vi "test_DAC_IO.vi"() -> ()   [LabVIEW 2019]
uses:
  <vilib>/DAQmx/write.llb/DAQmx Write (Analog Wfm 1Chan NSamp).vi
  <vilib>/DAQmx/read.llb/DAQmx Read (Analog DBL 1Chan 1Samp).vi
  <vilib>/DAQmx/create/channels.llb/DAQmx Create Channel (AO-Voltage-Basic).vi
  <vilib>/DAQmx/configure/timing.llb/DAQmx Timing (Use Waveform).vi
  <vilib>/DAQmx/miscellaneous.llb/DAQmx Fill In Error Info.vi
  <vilib>/DAQmx/create/channels.llb/DAQmx Create Channel (AI-Voltage-Basic).vi
  <vilib>/DAQmx/configure/timing.llb/DAQmx Timing (Sample Clock).vi
panel:
  in  "auto_stop":bool
  in  "stop":bool
  out "wf_chart_in":dbl(graph)
  in  "rate_in":dbl=1000.0 format="%0.2f"
  in  "chan_in":tag
  out "message":string
  out "wf_graph_out":waveform(dbl)(graph)
  in  "waveform":T1(ring)
  in  "N_steps":i32=100
  in  "T_sweep":dbl=1.0
  in  "N_sweeps":i32=2
  in  "chan_out":tag="Dev1/ao0"
  # "s"
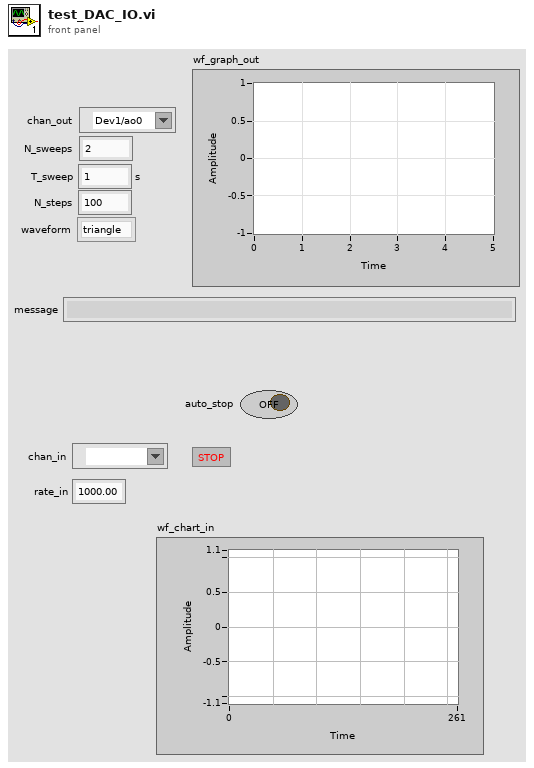
[diagram p1: front panel]
types:
  T1 = enum16{"triangle", "saw_direct", "saw_invert", "sine"}
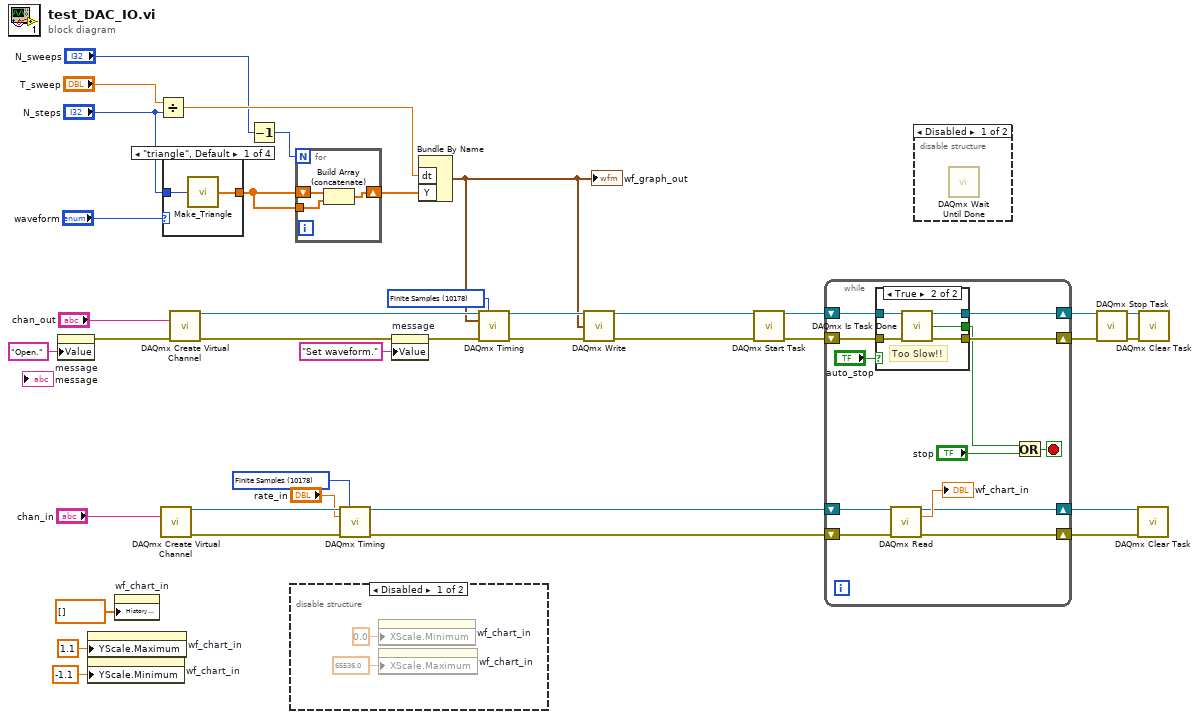
[diagram p0: block diagram]
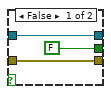
[diagram p4: hidden frame]
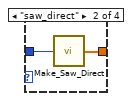
[diagram p5: hidden frame]
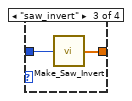
[diagram p6: hidden frame]
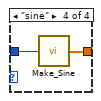
[diagram p7: hidden frame]
diagram:
  w11 = 10178 items=["Finite Samples"=10178, "Continuous Samples"=10123, "Hardware Timed Single Point"=12522] ("sample mode")
  w38 = 10178 items=["Finite Samples"=10178, "Continuous Samples"=10123, "Hardware Timed Single Point"=12522] ("sample mode")
  n1 = property on="message" class="Str"("Value"="Open." ("message")) -> (error out=w22:errorcluster)  [unwired: 2 in, 1 out]
  n2 = property on="wf_chart_in" class="WFChart (strict)"("YScale.Maximum"=1.1 ("Y Scale.Range:Maximum")) -> ()  [unwired: 2 in, 2 out]
  n3 = property on="wf_chart_in" class="WFChart (strict)"("YScale.Minimum"=-1.1 ("Y Scale.Range:Minimum")) -> ()  [unwired: 2 in, 2 out]
  n4 = property on="wf_chart_in" class="WFChart (strict)"("History Data"=dbl[] []) -> ()  [unwired: 2 in, 2 out]
  n5 = Divide(x="T_sweep", y="N_steps") -> (x/y=w29:dbl)
  n6 = call-poly <vilib>:"DAQmx Create Virtual Channel.vi"("physical channels"="chan_in") -> ("task out"=w15:refnum<k21>, "error out"=w13:errorcluster)  [unwired: 13 in]
  n7 = case shown="\"triangle\", Default" "waveform" {
    tunnel: "N_steps" -> [w41 w43 w45 w47]
    tunnel: [w40 w42 w44 w46] -> w30
    frame "triangle", Default {
      n8 = call "Make_Triangle.vi"("N_steps_1"=w41) -> ("TriangleWaveform"=w40:dbl[])
    }
    frame "saw_direct" {
      n9 = call "Make_Saw_Direct.vi"("N_steps_1"=w43) -> ("SawDirectWaveform"=w42:dbl[])
    }
    frame "saw_invert" {
      n10 = call "Make_Saw_Invert.vi"("N_steps_1"=w45) -> ("SawInvertWaveform"=w44:dbl[])
    }
    frame "sine" {
      n11 = call "Make_Sine.vi"("N_steps_1"=w47) -> ("SineWaveform"=w46:dbl[])
    }
  }
  n12 = call-poly <vilib>:"DAQmx Create Virtual Channel.vi"("physical channels"="chan_out", "error in"=w22) -> ("task out"=w32:refnum<k21>, "error out"=w20:errorcluster)  [unwired: 12 in]
  n13 = Decrement(x="N_sweeps") -> (x-1=w28:i32)
  n14 = disable-structure shown="Disabled" {
    frame Disabled {
      n15 = property on="wf_chart_in" class="WFChart (strict)"("XScale.Minimum"=0.0 ("X Scale.Range:Minimum")) -> ()  [unwired: 2 in, 2 out]
      n16 = property on="wf_chart_in" class="WFChart (strict)"("XScale.Maximum"=65536.0 ("X Scale.Range:Maximum")) -> ()  [unwired: 2 in, 2 out]
    }
    frame Enabled {
    }
  }
  n17 = for {
    N: w28 -> [_]
    shift-right: [w50] -> w31
    shift-left: w30 -> [w52]
    tunnel: w30 -> [w51]
    n18 = Build Array (concatenate)(w52, w51) -> (w50:dbl[])
  }
  n19 = call-poly <vilib>:"DAQmx Timing.vi"("task/channels in"=w15, "sample mode"=w11, "rate"="rate_in", "error in"=w13) -> ("task out"=w14:refnum<k21>, "error out"=w12:errorcluster)  [unwired: 10 in]
  n20 = property on="message" class="Str"(error in=w20, "Value"="Set waveform." ("message")) -> (error out=w19:errorcluster)  [unwired: 1 in, 1 out]
  n21 = Bundle By Name("dt"=w29, "Y"=w31) -> (w23:waveform(dbl))  [unwired: 1 in]
  "wf_graph_out" <- w23
  n22 = call-poly <vilib>:"DAQmx Timing.vi"("task/channels in"=w32, "sample mode"=w38, "waveform"=w23, "error in"=w19) -> ("task out"=w34:refnum<k21>, "error out"=w33:errorcluster)  [unwired: 10 in]
  n23 = call-poly <vilib>:"DAQmx Write.vi"("task/channels in"=w34, "data"=w23, "error in"=w33) -> ("task out"=w35:refnum<k21>, "error out"=w17:errorcluster)  [unwired: 10 in, 1 out]
  n24 = call <vilib>:"DAQmx Start Task.vi"("task/channels in"=w35, "error in"=w17) -> ("task out"=w4:refnum<k21>, "error out"=w3:errorcluster)  [unwired: 12 in]
  n25 = while {
    shift-right: [w62] -> w9
    shift-left: w14 -> [w65]
    shift-right: [w61] -> w8
    shift-left: w12 -> [w64]
    shift-right: [w56] -> w2
    shift-left: w4 -> [w57]
    shift-right: [w54] -> w1
    shift-left: w3 -> [w55]
    stop <- w60 stop-if-true
    n26 = case shown="True" "auto_stop" {
      tunnel: [FALSE ("x") w73] -> w53
      tunnel: w57 -> [w68 w72]
      tunnel: [w68 w71] -> w56
      tunnel: w55 -> [w66 w70]
      tunnel: [w66 w69] -> w54
      frame False {
      }
      frame True {
        # "Too Slow!!"
        n27 = call <vilib>:"DAQmx Is Task Done.vi"("task/channels in"=w72, "error in"=w70) -> ("task out"=w71:refnum<k21>, "task done?"=w73:bool, "error out"=w69:errorcluster)  [unwired: 11 in]
      }
    }
    n28 = call-poly <vilib>:"DAQmx Read.vi"("task/channels in"=w65, "error in"=w64) -> ("task out"=w62:refnum<k21>, "data"=→"wf_chart_in":dbl, "error out"=w61:errorcluster)  [unwired: 11 in]
    n29 = Or(x=w53, y="stop") -> (x .or. y?=w60:bool)
  }
  n30 = disable-structure shown="Disabled" {
    frame Disabled {
      n31 = call <vilib>:"DAQmx Wait Until Done.vi"() -> ()  [unwired: 14 in, 2 out]
    }
    frame Enabled {
    }
  }
  n32 = call <vilib>:"DAQmx Stop Task.vi"("task/channels in"=w2, "error in"=w1) -> ("task out"=w37:refnum<k21>, "error out"=w36:errorcluster)  [unwired: 12 in]
  n33 = call <vilib>:"DAQmx Clear Task.vi"("task in"=w9, "error in"=w8) -> ()  [unwired: 13 in, 1 out]
  n34 = call <vilib>:"DAQmx Clear Task.vi"("task in"=w37, "error in"=w36) -> ()  [unwired: 13 in, 1 out]
